vi "verify acquisition parameters in range.vi"(8 "error in (no error)":errorcluster, 11 "Simulated_CCD_Camera in":refnum<class "Simulated_CCD_Camera.lvclass">) -> (0 "error out":errorcluster, 3 "Simulated_CCD_Camera out":refnum<class "Simulated_CCD_Camera.lvclass">)   [LabVIEW 2018, in "Simulated_CCD_Camera.lvclass"]
doc: "Verify if the parameters of the camera are in range\n\nThe operating parameters of the CCDs must be within a predefined range. This function verifies if the values provided for these parameters meet this specification. If not, ACS will not allow to start an exposure."
uses:
  Simulated_CCD_Camera.lvclass
  Simulated_CCD_Camera.lvclass/Simulated_CCD_Camera.ctl
panel:
  out "New SET parameters 2":T1
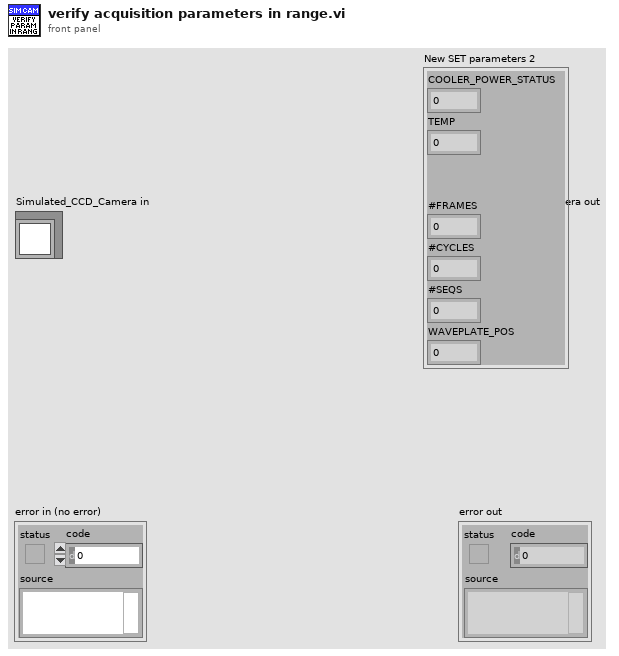
[diagram p1: front panel]
types:
  T1 = cluster{"COOLER_POWER_STATUS":u16, "TEMP":i32, "#FRAMES":u32, "#CYCLES":u32, "#SEQS":u32, "WAVEPLATE_POS":u16}
  T2 = cluster{"COOLER_POWER_STATUS":u16, "TEMP":i32, "EXPTIME":dbl, "#FRAMES":u32, "#CYCLES":u32, "#SEQS":u32, "WAVEPLATE_POS":u16}
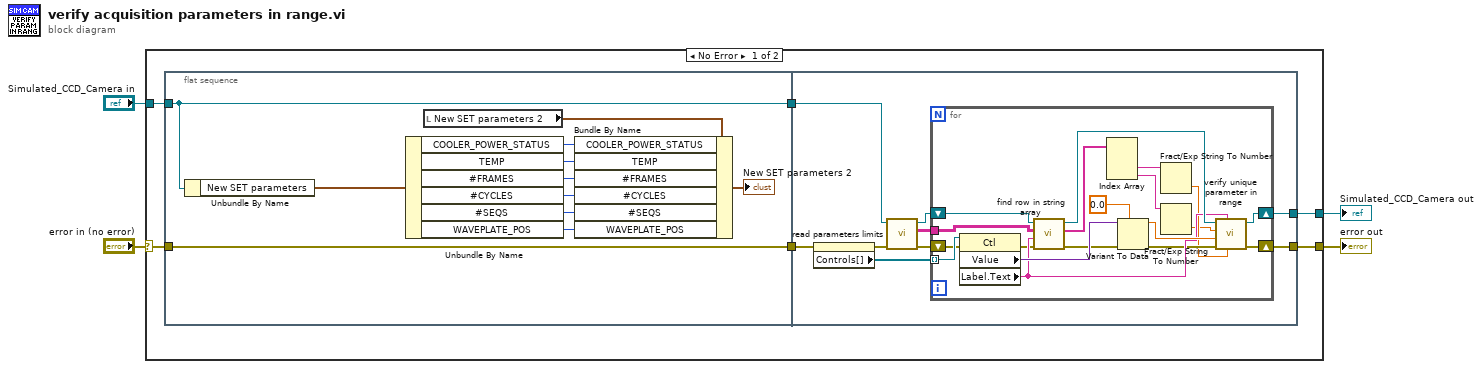
[diagram p0: block diagram]
diagram:
  n1 = case shown="No Error" "error in (no error)" {
    selector: "error in (no error)" -> [w8 w51]
    tunnel: [w10 w51] -> w3
    tunnel: [w9 w50] -> w2
    tunnel: "Simulated_CCD_Camera in" -> [w7 w50]
    frame No Error {
      n2 = flat-sequence {
        tunnel: w7 -> [w20]
        tunnel: w8 -> [w21]
        tunnel: [w21] -> w6
        tunnel: [w20] -> w5
        tunnel: [w30] -> w10
        tunnel: [w29] -> w9
        tunnel: w6 -> [w23]
        tunnel: w5 -> [w25]
        frame #0 {
          n3 = Unbundle By Name(w20) -> ("New SET parameters"=w17:T2)
          n4 = Unbundle By Name(w17) -> ("COOLER_POWER_STATUS"=w16:u16, "TEMP"=w15:i32, "#FRAMES"=w14:u32, "#CYCLES"=w13:u32, "#SEQS"=w12:u32, "WAVEPLATE_POS"=w11:u16)
          n5 = local read "New SET parameters 2"() -> (w19:T1)
          n6 = Bundle By Name(cluster=w19, "COOLER_POWER_STATUS"=w16, "TEMP"=w15, "#FRAMES"=w14, "#CYCLES"=w13, "#SEQS"=w12, "WAVEPLATE_POS"=w11) -> (→"New SET parameters 2":T1)
        }
        frame #1 {
          n7 = property on="New SET parameters 2" class="Clust (strict)"(error in=w23) -> (error out=w22:errorcluster, "Controls[]"=w24:refnum<vi>[])  [unwired: 1 in, 1 out]
          n8 = call "read parameters limits.vi"("error in (no error)"=w22, "Simulated_CCD_Camera in"=w25) -> ("error out"=w28:errorcluster, "limit values spreadsheet"=w27:string[][], "Simulated_CCD_Camera out"=w26:refnum<class "Simulated_CCD_Camera.lvclass">)  [unwired: 7 in]
          n9 = for {
            shift-right: [w49] -> w30
            shift-left: w28 -> [w33]
            tunnel: w24 -> [w48] mode=indexing
            tunnel: w27 -> [w43]
            shift-right: [w44] -> w29
            shift-left: w26 -> [w41]
            n10 = property class="Ctl"(reference=w48, error in=w33) -> (error out=w35:errorcluster, "Value"=w47:variant, "Label.Text"=w37:string)  [unwired: 1 out]
            n11 = call "find row in string array.vi"("error in (no error)"=w35, "parameter name"=w37, "limit values"=w43, "Simulated_CCD_Camera in"=w41) -> ("error out"=w34:errorcluster, "row"=w42:string[], "Simulated_CCD_Camera out"=w40:refnum<class "Simulated_CCD_Camera.lvclass">)  [unwired: 5 in]
            n12 = Index Array(array=w42) -> (element #2=w39:string, element #3=w38:string)  [unwired: 3 in, 1 out]
            n13 = Variant To Data(error in=w34, type=0.0, Variant=w47) -> (data=w45:dbl, error out=w36:errorcluster)
            n14 = Fract/Exp String To Number(string=w39) -> (number=w32:dbl)  [unwired: 3 in, 1 out]
            n15 = Fract/Exp String To Number(string=w38) -> (number=w31:dbl)  [unwired: 3 in, 1 out]
            n16 = call "verify unique parameter in range.vi"("lower limit"=w32, "parameter name"=w37, "error in (no error)"=w36, "value"=w45, "upper limit"=w31, "Simulated_CCD_Camera in"=w40) -> ("error out"=w49:errorcluster, "Simulated_CCD_Camera out"=w44:refnum<class "Simulated_CCD_Camera.lvclass">)  [unwired: 4 in]
          }
        }
      }
    }
    frame Error {
    }
  }
  "error out" <- w3
  "Simulated_CCD_Camera out" <- w2
